vi "HXGetDisplayName.vi"(11 "String":string) -> (3 "String 2":string)   [LabVIEW 2020]
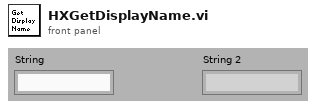
[diagram p1: front panel]
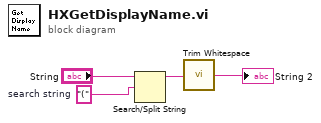
[diagram p0: block diagram]
diagram:
  w3 = "("  # search string
  n1 = Search/Split String(string="String", search string/char (-)=w3) -> (substring before match=w2:string)  [unwired: 1 in, 2 out]
  n2 = call <vilib>:"Trim Whitespace.vi"("string"=w2) -> ("trimmed string"=→"String 2":string)  [unwired: 1 in]
